vi "ProgressBarExample.vi"() -> ()   [LabVIEW 2013]
doc: "This example shows how to implement a progress bar by calling a VI dynamically. \n\nThe example generates 3000 random numbers and a progress bar shows how far the generation has advanced. The generated numbers are put in the Data array at the end. \n\nThe progress bar is implemented with three subVIs that launch, update, and finally close it. This set of VIs is useful in large applications where progress bars maybe required in different components of the application. A custom message can be provided for the progress bar in each case."
panel:
  out "Data":dbl[](array[numeric]) format="%.2f"
  out "Current number":dbl format="%.2f"
  # "Select Help»Show Context Help and move the cursor \nover the VI icon to display help for this VI."
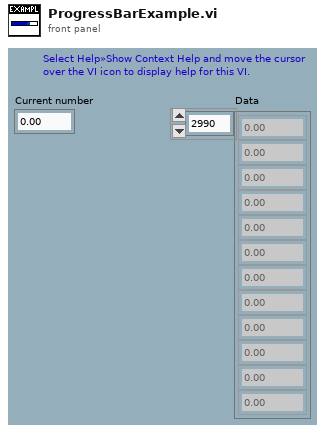
[diagram p1: front panel]
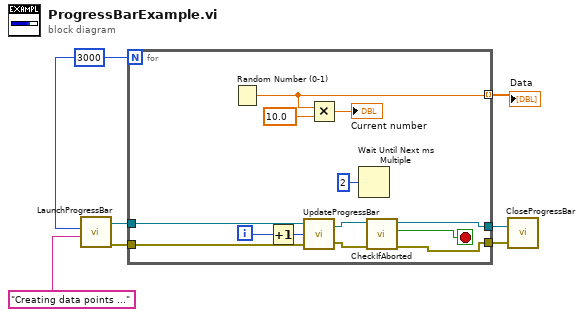
[diagram p0: block diagram]
diagram:
  w3 = 3000
  n1 = call "LaunchProgressBar.vi"("Title"="Creating data points ...", "MaxRange"=w3) -> ("error out"=w7:errorcluster, "reference out"=w6:refnum<vi>)  [unwired: 4 in]
  n2 = for {
    N: w3 -> [_]
    tunnel: [w17] -> w1 mode=indexing
    tunnel: w7 -> [w19]
    tunnel: w6 -> [w18]
    tunnel: [w8] -> w5
    tunnel: [w10] -> w4
    i -> [w20]
    stop <- w12 stop-if-true
    n3 = Random Number (0-1)() -> (number: 0 to 1=w17:dbl)
    n4 = Increment(x=w20) -> (x+1=w14:i32)
    n5 = call "UpdateProgressBar.vi"("error in"=w19, "PBarValue"=w14, "reference in"=w18) -> ("error out"=w9:errorcluster, "reference out"=w11:refnum<vi>)
    n6 = Multiply(x=w17, y=10.0) -> (x*y=→"Current number":dbl)
    n7 = Wait Until Next ms Multiple(millisecond multiple=u32 2) -> ()  [unwired: 1 out]
    n8 = call "CheckIfAborted.vi"("error in"=w9, "reference in"=w11) -> ("error out"=w8:errorcluster, "Abort?"=w12:bool, "reference out"=w10:refnum<vi>)  [unwired: 7 in]
  }
  "Data" <- w1
  n9 = call "CloseProgressBar.vi"("error in"=w5, "reference in"=w4) -> ()  [unwired: 1 out]
